vi "JSONtoArrayValue.vi"(8 "error in (no error)":errorcluster, 10 "data (parsed JSON)":T1(array[cluster]), 11 "Array in":refnum<vi>) -> (0 "error out":errorcluster, 3 "Variant":variant)   [LabVIEW 2019]
uses:
  <vilib>/Utility/Data Type/NI_Data Type.lvlib
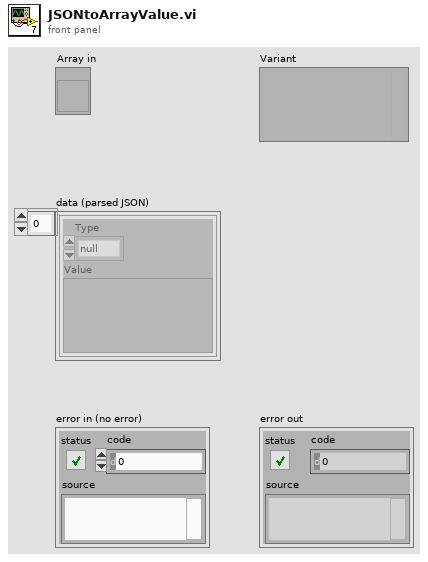
[diagram p1: front panel]
types:
  T1 = cluster{"Type":enum16{"null", "number", "boolean", "string", "array", "object", ""}, "Value":variant}[]
  T2 = enum16{"null", "number", "boolean", "string", "array", "object", ""}
  T3 = cluster{"Type":enum16{"null", "number", "boolean", "string", "array", "object", ""}, "Value":variant}
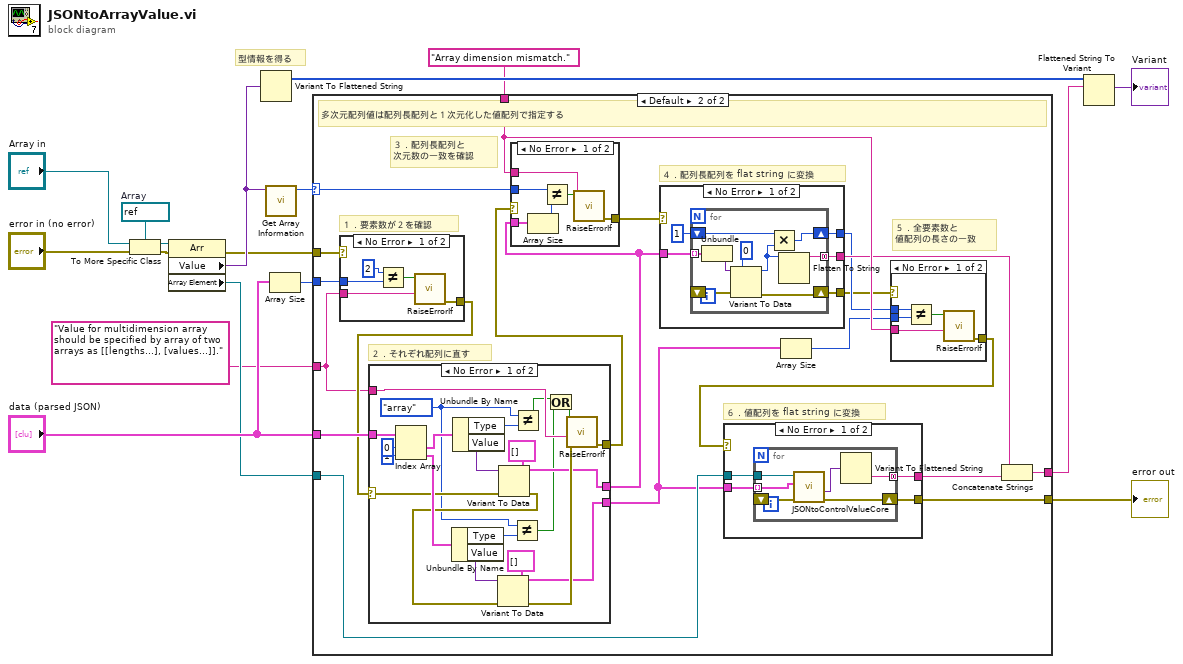
[diagram p0: block diagram]
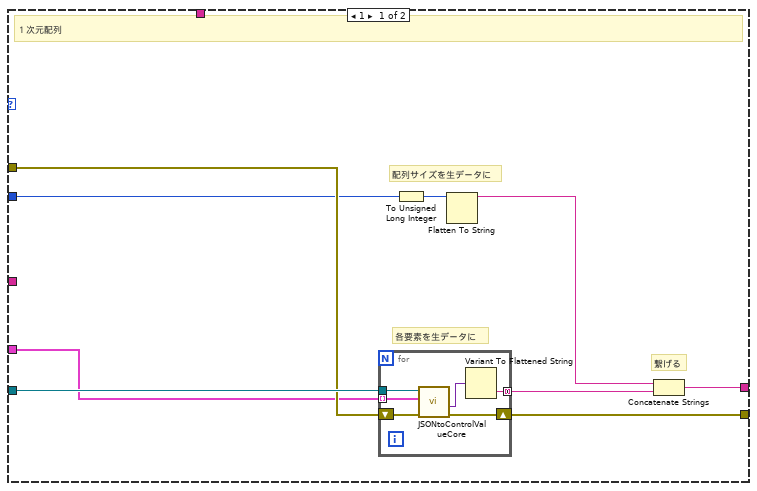
[diagram p2: hidden frame]
diagram:
  w4 = refnum<vi> refnum  # Array
  # "型情報を得る"
  n1 = To More Specific Class(target class=w4, reference="Array in", error in="error in (no error)") -> (specific class reference=w3:refnum<vi>, error out=w1:errorcluster)
  n2 = property class="Arr"(reference=w3, error in=w1) -> (error out=w11:errorcluster, "Value"=w14:variant, "Array Element"=w8:refnum<vi>)  [unwired: 1 out]
  n3 = Variant To Flattened String(Variant=w14) -> (1:w15:i16[])  [unwired: 1 out]
  n4 = call <vilib>:"Get Array Information.vi"("variant"=w14) -> ("number of dimensions"=w12:i32)  [unwired: 7 in, 3 out]
  n5 = Array Size(array="data (parsed JSON)") -> (size(s)=w17:i32)
  n6 = case shown="Default" w12 {
    selector: w12 -> [_ w49]
    tunnel: [w26 w52] -> w10
    tunnel: w8 -> [w25 w51]
    tunnel: w11 -> [w24 w35]
    tunnel: "data (parsed JSON)" -> [w23 w47]
    tunnel: [w19 w50] -> w13
    tunnel: w17 -> [w18 w40]
    tunnel: "Array dimension mismatch." ("error source (\" \")") -> [_ w48]
    tunnel: "Value for multidimension array should be specified by array of two arrays as [[lengths...], [values...]]." ("error source (\" \")") -> [_ w33]
    frame 1 {
      # "繋げる"
      # "各要素を生データに"
      # "配列サイズを生データに"
      # "１次元配列"
      n7 = for {
        tunnel: w25 -> [w32]
        shift-right: [w30] -> w26
        shift-left: w24 -> [w31]
        tunnel: w23 -> [w29] mode=indexing
        tunnel: [w27] -> w21 mode=concatenating
        n8 = call "JSONtoControlValueCore.vi"("error in"=w31, "Value"=w29, "Control in"=w32) -> ("error out"=w30:errorcluster, "Variant"=w28:variant)  [unwired: 7 in]
        n9 = Variant To Flattened String(Variant=w28) -> (data string=w27:string)  [unwired: 1 out]
      }
      n10 = To Unsigned Long Integer(number=w18) -> (unsigned 32bit integer=w22:u32)
      n11 = Flatten To String(anything=w22) -> (data string=w20:string)  [unwired: 3 in, 2 out]
      n12 = Concatenate Strings(w20, w21) -> (w19:string)
    }
    frame Default {
      # "６．値配列を flat string に変換"
      # "５．全要素数と\n値配列の長さの一致"
      # "４．配列長配列を flat string に変換"
      # "３．配列長配列と\n次元数の一致を確認"
      # "２．それぞれ配列に直す"
      # "１．要素数が２を確認"
      # "多次元配列値は配列長配列と１次元化した値配列で指定する"
      n13 = case shown="No Error" w35 {
        selector: w35 -> [_ w58]
        tunnel: w40 -> [w57 _]
        tunnel: [w54 w58] -> w39
        tunnel: w33 -> [w53 _]
        frame No Error {
          n14 = Not Equal?(x=2, y=w57) -> (x != y?=w55:bool)
          n15 = call "RaiseErrorIf.vi"("error message"=w53, "error? (true)"=w55) -> ("error out"=w54:errorcluster)  [unwired: 9 in]
        }
        frame Error {
        }
      }
      n16 = case shown="No Error" w39 {
        selector: w39 -> [w106 w120]
        tunnel: w47 -> [w111 _]
        tunnel: [w101 _] -> w42
        tunnel: [w100 _] -> w41
        tunnel: w33 -> [w119 _]
        tunnel: [w118 w120] -> w34
        frame No Error {
          w104 = T2."array" ("Type")
          n17 = Index Array(array=w111, index #1=0 ("index"), index #2=1 ("index")) -> (element #1=w108:T3, element #2=w107:T3)
          n18 = Unbundle By Name(w107) -> ("Type"=w114:T2, "Value"=w113:variant)
          n19 = Unbundle By Name(w108) -> ("Type"=w117:T2, "Value"=w116:variant)
          n20 = Variant To Data(error in=w106, type=T1 [], Variant=w116) -> (data=w101:T1, error out=w105:errorcluster)
          n21 = Variant To Data(error in=w105, type=T1 [], Variant=w113) -> (data=w100:T1, error out=w103:errorcluster)
          n22 = Not Equal?(x=w104, y=w114) -> (x != y?=w99:bool)
          n23 = Not Equal?(x=w104, y=w117) -> (x != y?=w98:bool)
          n24 = Or(x=w98, y=w99) -> (x .or. y?=w102:bool)
          n25 = call "RaiseErrorIf.vi"("error in (no error)"=w103, "error message"=w119, "error? (true)"=w102) -> ("error out"=w118:errorcluster)  [unwired: 8 in]
        }
        frame Error {
        }
      }
      n26 = case shown="No Error" w34 {
        selector: w34 -> [_ w97]
        tunnel: w49 -> [w91 _]
        tunnel: w48 -> [w96 _]
        tunnel: [w94 w97] -> w38
        tunnel: w42 -> [w93 _]
        frame No Error {
          n27 = Array Size(array=w93) -> (size(s)=w92:i32)
          n28 = Not Equal?(x=w91, y=w92) -> (x != y?=w95:bool)
          n29 = call "RaiseErrorIf.vi"("error message"=w96, "error? (true)"=w95) -> ("error out"=w94:errorcluster)  [unwired: 9 in]
        }
        frame Error {
        }
      }
      n30 = case shown="No Error" w38 {
        selector: w38 -> [_ w90]
        tunnel: [w80 _] -> w45
        tunnel: [w78 _] -> w43
        tunnel: [w77 w90] -> w37
        tunnel: w42 -> [w76 _]
        frame No Error {
          n31 = for {
            tunnel: [w89] -> w80 mode=concatenating
            tunnel: w76 -> [w88] mode=indexing
            shift-right: [w83] -> w78
            shift-left: u32 1 -> [w85]
            shift-right: [w81] -> w77
            shift-left: _ -> [w82]
            n32 = Unbundle(w88) -> ("Value"=w87:variant)  [unwired: 1 out]
            n33 = Variant To Data(error in=w82, type=u32 0, Variant=w87) -> (data=w84:u32, error out=w81:errorcluster)
            n34 = Multiply(x=w85, y=w84) -> (x*y=w83:u32)
            n35 = Flatten To String(anything=w84) -> (data string=w89:string)  [unwired: 3 in, 2 out]
          }
        }
        frame Error {
        }
      }
      n36 = Array Size(array=w41) -> (size(s)=w44:i32)
      n37 = case shown="No Error" w37 {
        selector: w37 -> [_ w75]
        tunnel: w48 -> [w74 _]
        tunnel: w44 -> [w73 _]
        tunnel: w43 -> [w72 _]
        tunnel: [w70 w75] -> w36
        frame No Error {
          n38 = Not Equal?(x=w72, y=w73) -> (x != y?=w71:bool)
          n39 = call "RaiseErrorIf.vi"("error message"=w74, "error? (true)"=w71) -> ("error out"=w70:errorcluster)  [unwired: 9 in]
        }
        frame Error {
        }
      }
      n40 = case shown="No Error" w36 {
        selector: w36 -> [_ w69]
        tunnel: [w62 w69] -> w52
        tunnel: w51 -> [w61 _]
        tunnel: [w60 _] -> w46
        tunnel: w41 -> [w59 _]
        frame No Error {
          n41 = for {
            tunnel: w61 -> [w68]
            shift-right: [w66] -> w62
            shift-left: _ -> [w67]
            tunnel: [w64] -> w60 mode=concatenating
            tunnel: w59 -> [w63] mode=indexing
            n42 = call "JSONtoControlValueCore.vi"("error in"=w67, "Value"=w63, "Control in"=w68) -> ("error out"=w66:errorcluster, "Variant"=w65:variant)  [unwired: 7 in]
            n43 = Variant To Flattened String(Variant=w65) -> (data string=w64:string)  [unwired: 1 out]
          }
        }
        frame Error {
        }
      }
      n44 = Concatenate Strings(w45, w46) -> (w50:string)
    }
  }
  "error out" <- w10
  n45 = Flattened String To Variant(6:w13, 7:w15) -> (3:→"Variant":variant)  [unwired: 1 in, 1 out]
